vi "main.vi"() -> ()   [LabVIEW 2021]
uses:
  <vilib>/Analysis/NI_AAL_SigProc.lvlib
  <vilib>/Analysis/NI_AALBase.lvlib
panel:
  out "size(s) 2":i32
  in  "intervals":i32=10
  out "X Values":dbl[](array[numeric]) format="%0.2f"
  out "Histogram Graph":T1(graph)
  out "size(s)":i32
  out "Amplitudes":dbl[](array[numeric])
  out "Locations":dbl[](array[numeric])
  in  "threshold":dbl format="%0.2f"
  out "Signals 2":dynamicdata(graph) caption="Signals"
  in  "Filename":path=path "test.lvm"
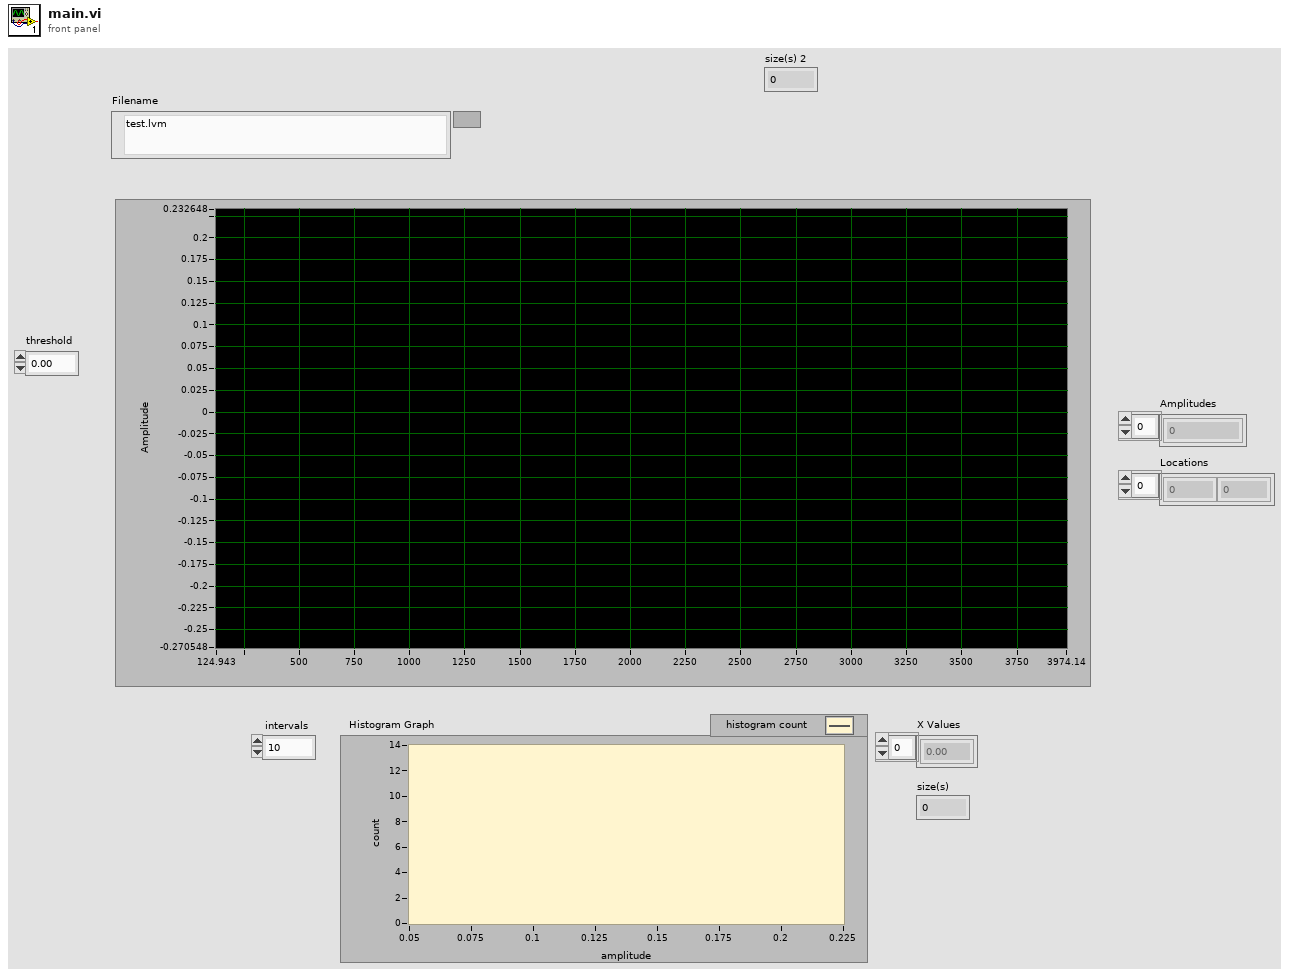
[diagram p1: front panel]
types:
  T1 = cluster{"X Values":dbl[], "Histogram: h(x)":i32[]}
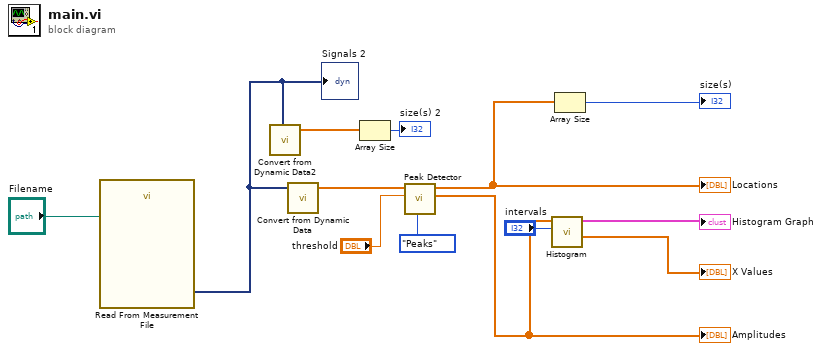
[diagram p0: block diagram]
diagram:
  n1 = call "Read From Measurement File"("Filename"="Filename") -> ("Signals"=w3:dynamicdata)  [unwired: 5 in, 5 out]
  "Signals 2" <- w3
  n2 = call "Convert from Dynamic Data2"("Dynamic Data Type"=w3) -> ("Array"=w2:dbl[])  [unwired: 3 in]
  n3 = call "Convert from Dynamic Data"("Dynamic Data Type"=w3) -> ("Array"=w12:dbl[])  [unwired: 3 in]
  n4 = Array Size(array=w2) -> (size(s)=→"size(s) 2":i32)
  n5 = call <vilib>:"Peak Detector.vi"("peaks/valleys"=enum32{"Peaks", "Valleys"}."Peaks", "threshold"="threshold", "X"=w12) -> ("Amplitudes"=w5:dbl[], "Locations"=w8:dbl[])  [unwired: 4 in, 3 out]
  "Locations" <- w8
  "Amplitudes" <- w5
  n6 = call <vilib>:"Histogram.vi"("intervals"="intervals", "X"=w5) -> ("X Values"=→"X Values":dbl[], "Histogram Graph"=→"Histogram Graph":T1)  [unwired: 6 in, 2 out]
  n7 = Array Size(array=w8) -> (size(s)=→"size(s)":i32)
